vi "GetHeader.vi"(11 "String in":string) -> (0 "Endian":T1(ring), 3 "String out":string, 5 "Title":string)   [LabVIEW 2022 SP3]
panel:
  out "Endian Indicator":string
  out "subsys data offset":string
  out "version":u16 format="%.0x"
  # "Field Value\nVersion When creating a MAT-file, set this field to 0x0100.\n\n\nEndian Indicator\nContains the two characters, M and I, written to the MAT-file in this order, as a 16-bit value. If, when read from the MAT-file as a 16-bit value, the characters appear in reversed order (IM rather than MI), it indicates that the program reading the MAT-file must perform byte-swapping to interpret the data in the MAT-file correctly."
  # "Header Subsystem Data Offset Field\nBytes 117 through 124 of the header contain an offset to subsystem-specific data in the MAT-file. All zeros or all spaces in this field indicate that there is no subsystem-specific data stored in the file."
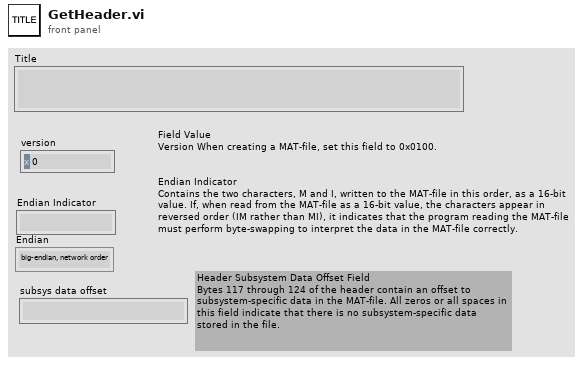
[diagram p1: front panel]
types:
  T1 = enum16{"big-endian, network order", "native, host order", "little-endian"}
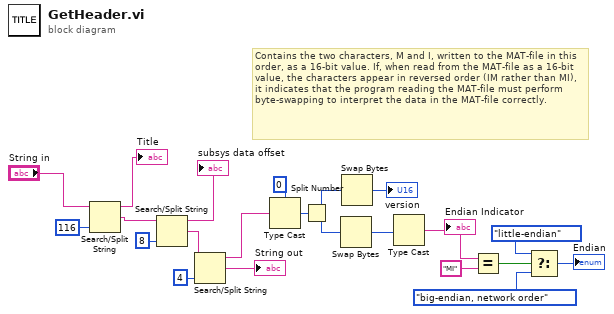
[diagram p0: block diagram]
diagram:
  # "Contains the two characters, M and I, written to the MAT-file in this order, as a 16-bit value. If, when read from the MAT-file as a 16-bit value, the characters appear in reversed order (IM rather than MI), it indicates that the program reading the MAT-file must perform byte-swapping to interpret the data in the MAT-file correctly."
  n1 = Search/Split String(string="String in", offset (0)=116) -> (substring before match=→"Title":string, match + rest of string=w10:string)  [unwired: 1 in, 1 out]
  n2 = Search/Split String(string=w10, offset (0)=8) -> (substring before match=→"subsys data offset":string, match + rest of string=w12:string)  [unwired: 1 in, 1 out]
  n3 = Search/Split String(string=w12, offset (0)=4) -> (substring before match=w15:string, match + rest of string=→"String out":string)  [unwired: 1 in, 1 out]
  n4 = Type Cast(type=u32 0 ("offset (0)"), x=w15) -> (*(type *) &x=w16:u32)
  n5 = Split Number(x=w16) -> (hi(x)=w21:u16, lo(x)=w20:u16)
  n6 = Swap Bytes(anything=w20) -> (byte swapped=w7:u16)
  n7 = Swap Bytes(anything=w21) -> (byte swapped=→"version":u16)
  n8 = Type Cast(x=w7) -> (*(type *) &x=w6:string)  [unwired: 1 in]
  "Endian Indicator" <- w6
  n9 = Equal?(x=w6, y="MI") -> (x = y?=w4:bool)
  n10 = Select(t=T1."little-endian" ("byte order"), s=w4, f=T1."big-endian, network order" ("byte order")) -> (s? t:f=→"Endian":T1)
